vi "InitSerial.vi"(8 "Serial Configuration 2":T1={"Baud Rate"=115200, "Parity"=0, "Data Bits"=7, "Stop Bits"=10, "Flow Control"=0} {"Flow Control" items=["None", "XON/XOFF", "RTS/CTS", "XON/XOFF & RTS/CTS", "DTR/DSR", "XON/XOFF & DTR/DSR"]; "Stop Bits" items=["1.0"=10, "1.5"=15, "2.0"=20]; "Data Bits" items=["7"=7, "8"=8]; "Parity" items=["None", "Odd", "Even", "Mark", "Space"]; "Baud Rate" items=["300"=300, "600"=600, "1200"=1200, "2400"=2400, "4800"=4800, "9600"=9600, "19200"=19200]}, 9 "error in (no error)":errorcluster, 10 "ID Query (True)":bool=TRUE, 11 "VISA resource name":refnum<visa-resource-name>) -> (1 "VISA resource name out":refnum<visa-resource-name>, 3 "error out":errorcluster)   [LabVIEW 2024]
panel:
  # "EDIT: Serial settings must match those on the physical instrument.  Review user's manual to determine the correct Flow Control protocol for the instrument.  \"None\" is the least robust option for this setting, and could lead to unreliable data transmission."
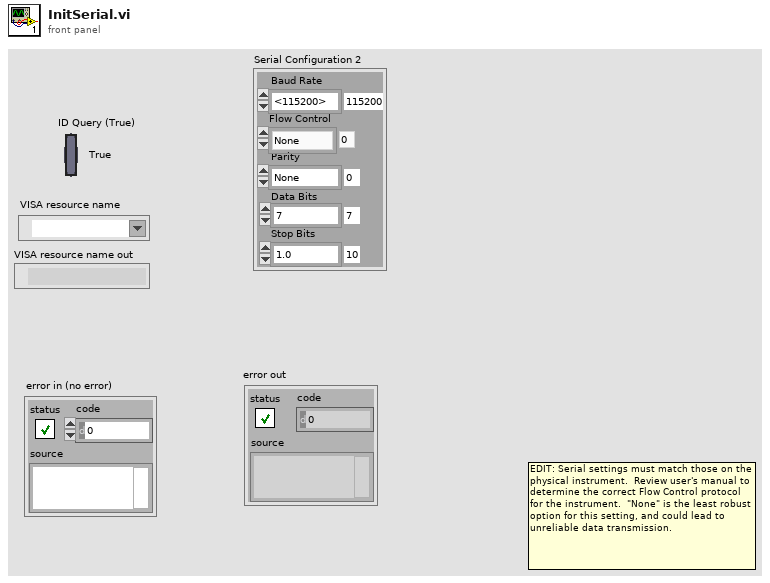
[diagram p1: front panel]
types:
  T1 = cluster{"Baud Rate":u32, "Parity":u16, "Data Bits":u16, "Stop Bits":u16, "Flow Control":u16}
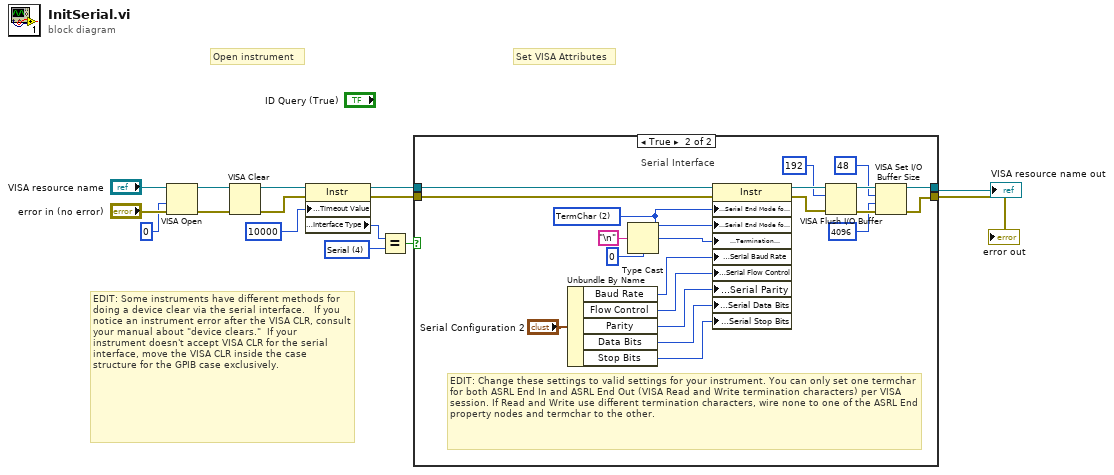
[diagram p0: block diagram]
diagram:
  w8 = u16 4 items=["GPIB"=1, "VXI"=2, "GPIB-VXI"=3, "Serial"=4, "PXI"=5, "TCPIP"=6, "USB"=7] ("Interface Information:Interface Type")
  # "EDIT: Some instruments have different methods for doing a device clear via the serial interface.   If you notice an instrument error after the VISA CLR, consult your manual about \"device clears.\"  If your instrument doesn't accept VISA CLR for the serial interface, move the VISA CLR inside the case  structure for the GPIB case exclusively."
  # "Set VISA Attributes"
  # "Open instrument"
  n1 = VISA Open(access mode=u32 0, error in (no error)="error in (no error)", VISA resource name="VISA resource name") -> (VISA resource name=w6:refnum<visa-resource-name>, error out=w5:errorcluster)  [unwired: 2 in]
  n2 = VISA Clear(VISA resource name=w6, error in (no error)=w5) -> (VISA resource name out=w4:refnum<visa-resource-name>, error out=w3:errorcluster)
  n3 = property class="Instr"(reference=w4, error in=w3, "General Settings:Timeout Value"=u32 10000) -> (reference out=w11:refnum<visa-resource-name>, error out=w10:errorcluster, "Interface Information:Interface Type"=w13:u16)
  n4 = Equal?(x=w13, y=w8) -> (x = y?=w9:bool)
  n5 = case shown="True" w9 {
    tunnel: [w16 w35] -> w2
    tunnel: [w17 w32] -> w1
    tunnel: w11 -> [w16 w37]
    tunnel: w10 -> [w17 w38]
    frame False {
      # "EDIT: Remove interfaces not supported by your instrument."
      # "GPIB, TCP/IP, and USB Interface"
    }
    frame True {
      w25 = u16 2 items=["None", "LastBit", "TermChar"] ("Serial Settings:Serial End Mode for Reads")
      # "EDIT: Change these settings to valid settings for your instrument. You can only set one termchar for both ASRL End In and ASRL End Out (VISA Read and Write termination characters) per VISA session. If Read and Write use different termination characters, wire none to one of the ASRL End property nodes and termchar to the other."
      # "Serial Interface"
      n6 = Unbundle By Name("Serial Configuration 2") -> ("Baud Rate"=w23:u32, "Flow Control"=w19:u16, "Parity"=w21:u16, "Data Bits"=w22:u16, "Stop Bits"=w18:u16)
      n7 = Type Cast(type=u8 0, x="\n" ("Line Feed Constant")) -> (*(type *) &x=w24:u8)
      n8 = property class="Instr"(reference=w37, error in=w38, "Serial Settings:Serial End Mode for Reads"=w25, "Serial Settings:Serial End Mode for Writes"=w25, "Message Based Settings:Termination Character"=w24, "Serial Settings:Serial Baud Rate"=w23, "Serial Settings:Serial Flow Control"=w19, "Serial Settings:Serial Parity"=w21, "Serial Settings:Serial Data Bits"=w22, "Serial Settings:Serial Stop Bits"=w18) -> (reference out=w31:refnum<visa-resource-name>, error out=w34:errorcluster)
      n9 = VISA Flush I/O Buffer(VISA resource name=w31, mask (16)=u16 192, error in (no error)=w34) -> (VISA resource name out=w36:refnum<visa-resource-name>, error out=w33:errorcluster)
      n10 = VISA Set I/O Buffer Size(VISA resource name=w36, mask (16)=u16 48, size (4096)=u32 4096 ("size (0)"), error in (no error)=w33) -> (VISA resource name out=w35:refnum<visa-resource-name>, error out=w32:errorcluster)
    }
  }
  "VISA resource name out" <- w2
  "error out" <- w1
